vi "Write paramHigh.vi"(8 "error in (no error)":errorcluster, 10 "paramHigh":u16, 11 "ApplicationEvent in":refnum<class "ApplicationEvent.lvclass">) -> (0 "error out":errorcluster, 3 "ApplicationEvent out":refnum<class "ApplicationEvent.lvclass">)   [LabVIEW 2013, in "HardwareCharacterization.lvlib" / "ApplicationEvent.lvclass"]
uses:
  ApplicationEvent.lvclass
  ApplicationEvent.lvclass/ApplicationEvent.ctl
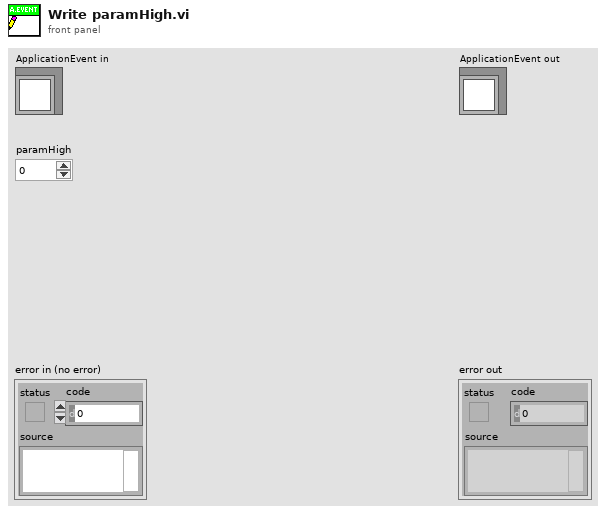
[diagram p1: front panel]
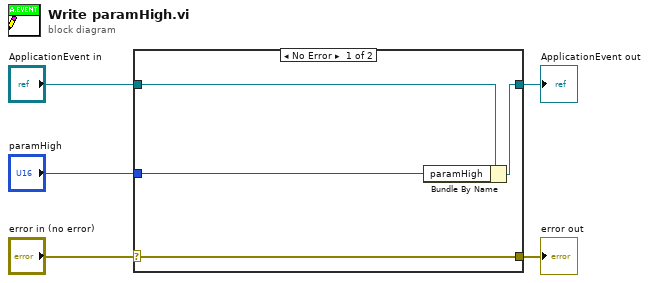
[diagram p0: block diagram]
diagram:
  n1 = case shown="No Error" "error in (no error)" {
    selector: "error in (no error)" -> [w9 w10]
    tunnel: [w9 w10] -> w4
    tunnel: [w7 w11] -> w2
    tunnel: "ApplicationEvent in" -> [w8 w11]
    tunnel: "paramHigh" -> [w6 _]
    frame No Error {
      n2 = Bundle By Name(cluster=w8, "paramHigh"=w6) -> (w7:refnum<class "ApplicationEvent.lvclass">)
    }
    frame Error {
    }
  }
  "error out" <- w4
  "ApplicationEvent out" <- w2
